vi "Convert Absolute Path to Relative Path from Application.vi"(8 "error in (no error)":errorcluster, 11 "Absolute Path":path) -> (0 "error out":errorcluster, 3 "Relative Path":path)   [LabVIEW 2020, in "File IO.lvlib"]
doc: "Converts a given absolute path to a relative path from the calling application."
uses:
  File IO.lvlib
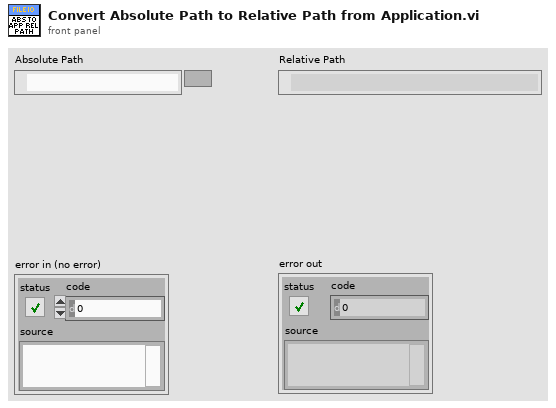
[diagram p1: front panel]
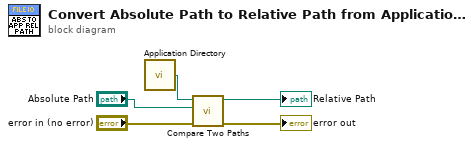
[diagram p0: block diagram]
diagram:
  n1 = call <vilib>:"Application Directory.vi"() -> ("Application Directory"=w2:path)
  n2 = call <vilib>:"Compare Two Paths.vi"("error in (no error)"="error in (no error)", "Path 2"="Absolute Path", "Path 1"=w2) -> ("error out"=→"error out":errorcluster, "Relative Path from 1 to 2"=→"Relative Path":path)  [unwired: 5 in, 2 out]
